vi "Login.vi"() -> ()   [LabVIEW 2013]
uses:
  <vilib>/Utility/miscctls.llb/LVPointTypeDef.ctl
  Globals/Global VI.vi
panel:
  in  "Cancel":bool
  in  "OK":bool
  in  "Password":string
  in  "Username":string
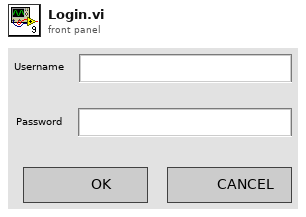
[diagram p1: front panel]
types:
  T1 = typedef "LVPointTypeDef.ctl" = cluster{"Horizontal":i16, "Vertical":i16}
  T2 = enum16{"Always On", "Always Off", "Off While Running"}
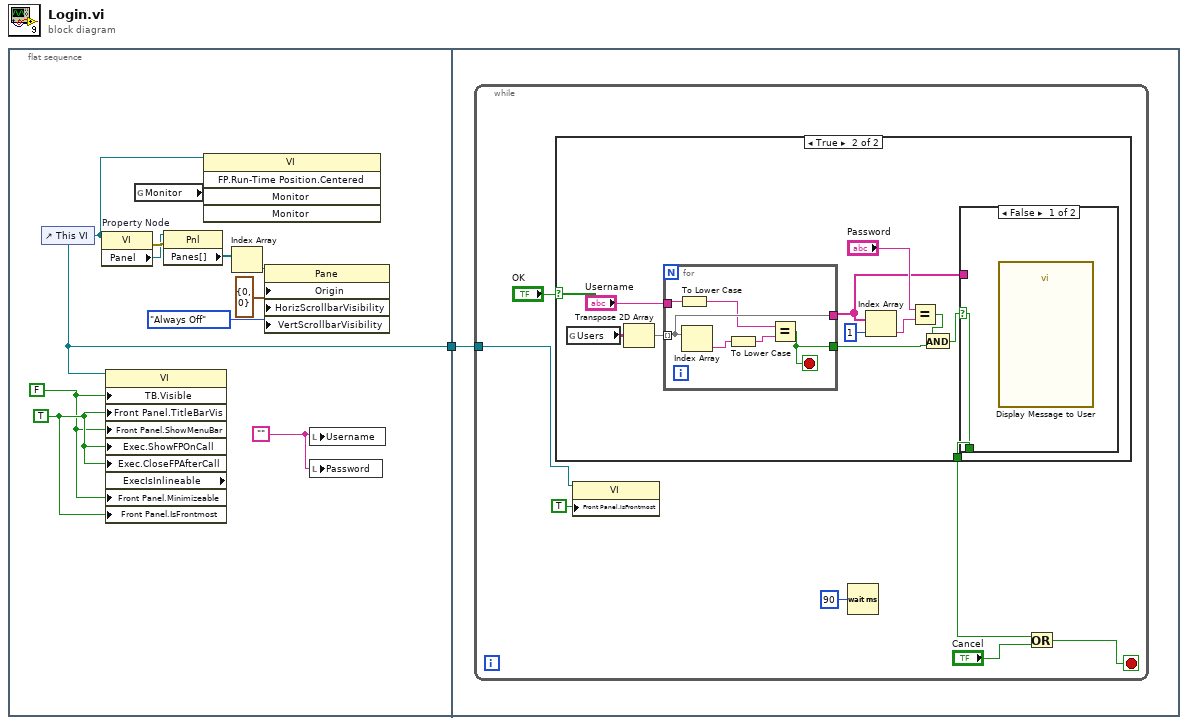
[diagram p0: block diagram]
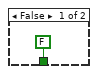
[diagram p2: hidden frame]
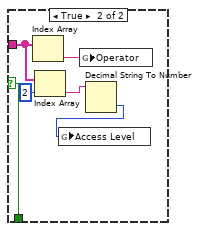
[diagram p3: hidden frame]
diagram:
  n1 = flat-sequence {
    tunnel: [w2] -> w1
    tunnel: w1 -> [w13]
    frame #0 {
      w4 = TRUE ("Tool Bar:Visible")
      w3 = FALSE ("Tool Bar:Visible")
      w6 = ""
      w7 = T2."Always Off" ("Horizontal Scrollbar Visibility")
      n2 = control-ref of="This VI"() -> (w2:refnum<vi>)
      n3 = property on="Property Node" class="VI"(reference=w2) -> (error out=w9:errorcluster, "Panel"=w8:refnum<vi>)  [unwired: 1 in, 1 out]
      n4 = property class="VI" props=["TB.Visible", "Front Panel.TitleBarVis", "Front Panel.ShowMenuBar", "Exec.ShowFPOnCall", "Exec.CloseFPAfterCall", "ExecIsInlineable", "Front Panel.Minimizeable", "Front Panel.IsFrontmost"](reference=w2, "TB.Visible"=w3, "Front Panel.TitleBarVis"=w4, "Front Panel.ShowMenuBar"=w3, "Exec.ShowFPOnCall"=w4, "Exec.CloseFPAfterCall"=w4, "Front Panel.Minimizeable"=w3, "Front Panel.IsFrontmost"=w4) -> ()  [unwired: 1 in, 3 out]
      n5 = global read "Global VI.vi" "Monitor"() -> (w5:u16)
      n6 = property class="Pnl"(reference=w8, error in=w9) -> ("Panes[]"=w10:refnum<vi>[])  [unwired: 2 out]
      n7 = invoke class="VI" method="FP.Run-Time Position.Centered"(reference=w2, "Monitor"=w5) -> ()  [unwired: 3 in, 5 out]
      n8 = Index Array "Index Array"(array=w10) -> (element=w11:refnum<vi>)  [unwired: 1 in]
      n9 = property class="Pane"(reference=w11, "Origin"=T1 {"Horizontal"=0, "Vertical"=0}, "HorizScrollbarVisibility"=w7, "VertScrollbarVisibility"=w7) -> ()  [unwired: 1 in, 2 out]
      n10 = local write "Username"(w6) -> ()
      n11 = local write "Password"(w6) -> ()
    }
    frame #1 {
      n12 = while {
        tunnel: w13 -> [w15]
        stop <- w20 stop-if-true
        n13 = case shown="True" "OK" {
          tunnel: [FALSE w27] -> w17
          frame False {
          }
          frame True {
            n14 = global read "Global VI.vi" "Users"() -> (w25:string[][])
            n15 = Transpose 2D Array(2D array=w25) -> (transposed array=w26:string[][])
            n16 = for {
              tunnel: w26 -> [w45] mode=indexing
              tunnel: "Username" -> [w43]
              tunnel: [w45] -> w28
              tunnel: [w44] -> w22
              stop <- w44 stop-if-true
              n17 = To Lower Case(string=w43) -> (all lower case string=w42:string)
              n18 = Index Array(array=w45) -> (element=w40:string)  [unwired: 1 in]
              n19 = To Lower Case(string=w40) -> (all lower case string=w41:string)
              n20 = Equal?(x=w42, y=w41) -> (x = y?=w44:bool)
            }
            n21 = Index Array(array=w28, index=1) -> (element=w30:string)
            n22 = Equal?(x="Password", y=w30) -> (x = y?=w24:bool)
            n23 = And(x=w24, y=w22) -> (x .and. y?=w23:bool)
            n24 = case shown="False" w23 {
              selector: w23 -> [w33 w38]
              tunnel: w28 -> [_ w37]
              tunnel: [w33 w38] -> w27
              frame False {
                n25 = call "Display Message to User"() -> ()  [unwired: 10 in, 2 out]
              }
              frame True {
                n26 = Index Array(array=w37) -> (element=w39:string)  [unwired: 1 in]
                n27 = Index Array(array=w37, index=2) -> (element=w35:string)
                n28 = global write "Global VI.vi" "Operator"(w39) -> ()
                n29 = Decimal String To Number(string=w35) -> (number=w34:i32)  [unwired: 2 in, 1 out]
                n30 = global write "Global VI.vi" "Access Level"(w34) -> ()
              }
            }
          }
        }
        n31 = property class="VI"(reference=w15, "Front Panel.IsFrontmost"=TRUE ("Front Panel Window:Is Frontmost")) -> ()  [unwired: 1 in, 2 out]
        n32 = Wait (ms)(milliseconds to wait=u32 90) -> ()  [unwired: 1 out]
        n33 = Or(x=w17, y="Cancel") -> (x .or. y?=w20:bool)
      }
    }
  }
